vi "sendUpdateCommand.vi"(8 "error in (no error)":errorcluster, 11 "Model in":refnum<class "Model.lvclass">) -> (0 "error out":errorcluster, 3 "Model out":refnum<class "Model.lvclass">)   [LabVIEW 2015, in "Model.lvclass"]
uses:
  Model.lvclass
  Typedefs/CommandSelector.ctl
  Model.lvclass/Model.ctl
  UserEvents/UserEvents.lvclass/UserEvents.ctl
  ICommandFactory/ICommandFactory.lvclass
  UserEvents/UserEvents.lvclass
  Typedefs/M1M3SSSTypedefs.lvlib
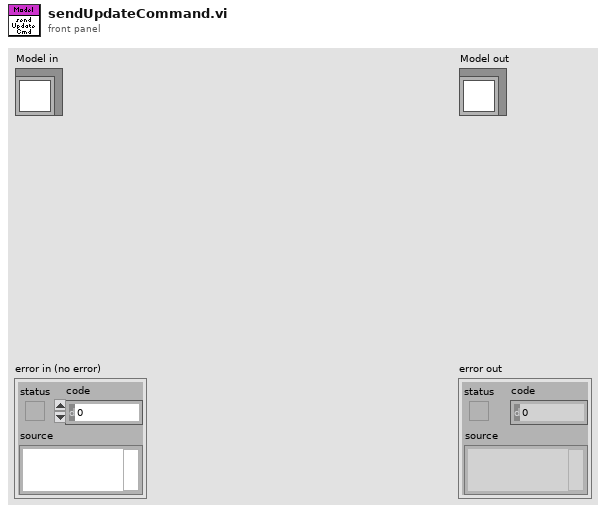
[diagram p1: front panel]
types:
  T1 = typedef "M1M3SSSTypedefs.lvlib/CommandSelector.ctl" = enum16{"ClearError", "Exit", "StandBy", "Start", "StartTest", "StopTest", "Update"}
  T2 = typedef "M1M3SSSTypedefs.lvlib/SubDataEvents.ctl" = cluster{"Command":refnum<user-event>}
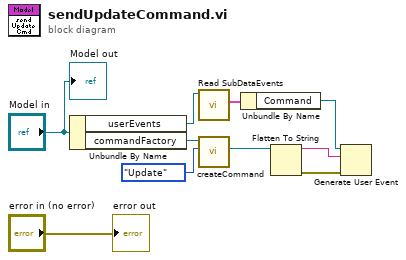
[diagram p0: block diagram]
diagram:
  n1 = Unbundle By Name("Model in") -> ("userEvents"=w3:refnum<class "UserEvents.lvclass">, "commandFactory"=w4:refnum<class "ICommandFactory.lvclass">)
  n2 = call "Read SubDataEvents.vi"("UserEvents in"=w3) -> ("SubDataEvents"=w9:T2)  [unwired: 9 in, 1 out]
  n3 = call-dynamic "createCommand.vi"("Command"=CommandSelector."Update", "ICommandFactory in"=w4) -> ("command"=w7:refnum<class "Command.lvclass">)  [unwired: 7 in, 2 out]
  n4 = Unbundle By Name(w9) -> ("Command"=w2:refnum<user-event>)
  n5 = Flatten To String(anything=w7) -> (data string=w6:string, error out=w1:errorcluster)  [unwired: 3 in, 1 out]
  n6 = Generate User Event(user event=w2, event data cluster=w6, error in=w1) -> ()  [unwired: 1 in, 2 out]
  "error out" <- "error in (no error)"
  "Model out" <- "Model in"
